vi "纳清蓝绿藻电极校准.vi"() -> ()   [LabVIEW 2016, in "斯坦道多参数.lvlib"]
uses:
  <vilib>/Utility/miscctls.llb/LVPointTypeDef.ctl
  <vilib>/Utility/miscctls.llb/LVPositionTypeDef.ctl
  <vilib>/Analysis/NI_AALBase.lvlib
panel:
  out "滤波设定":sgl
  in  "量程":u16(ring) items=["0-2000000", "0-200000"]
  out "第三点信号值":dbl
  out "第二点信号值":dbl
  out "第一点信号值":dbl
  out "报警信息":string
  out "通讯状态":string
  out "第三点校准值":dbl
  out "标液3":sgl
  out "第二点校准值":dbl
  out "第一点校准值":dbl
  in  "校准停止":bool
  in  "校准启动":bool
  in  "校准模式":u16(ring)=1 items=["两点校准", "单点校准", "三点校准"]
  out "最小值":sgl format="%#.2f"
  out "最大值":sgl format="%#.2f"
  out "波形图表":dbl(graph) caption="历史曲线"
  out "mean":dbl caption="均值" format="%#.2f"
  out "standard deviation":dbl caption="标准差" format="%#.2f"
  out "变异系数":dbl format="%#.6f"
  out "测量值":sgl format="%#.2f"
  out "提示":string
  out "标液2":sgl
  out "标液1":sgl
  out "原始光强数值":u16 caption="信号值"
  out "温度":dbl format="%#.2f"
  # "藻密度电极设定"
  # "℃"
  # "cells/mL"
  # "cells/mL"
  # "请选择校准模式:"
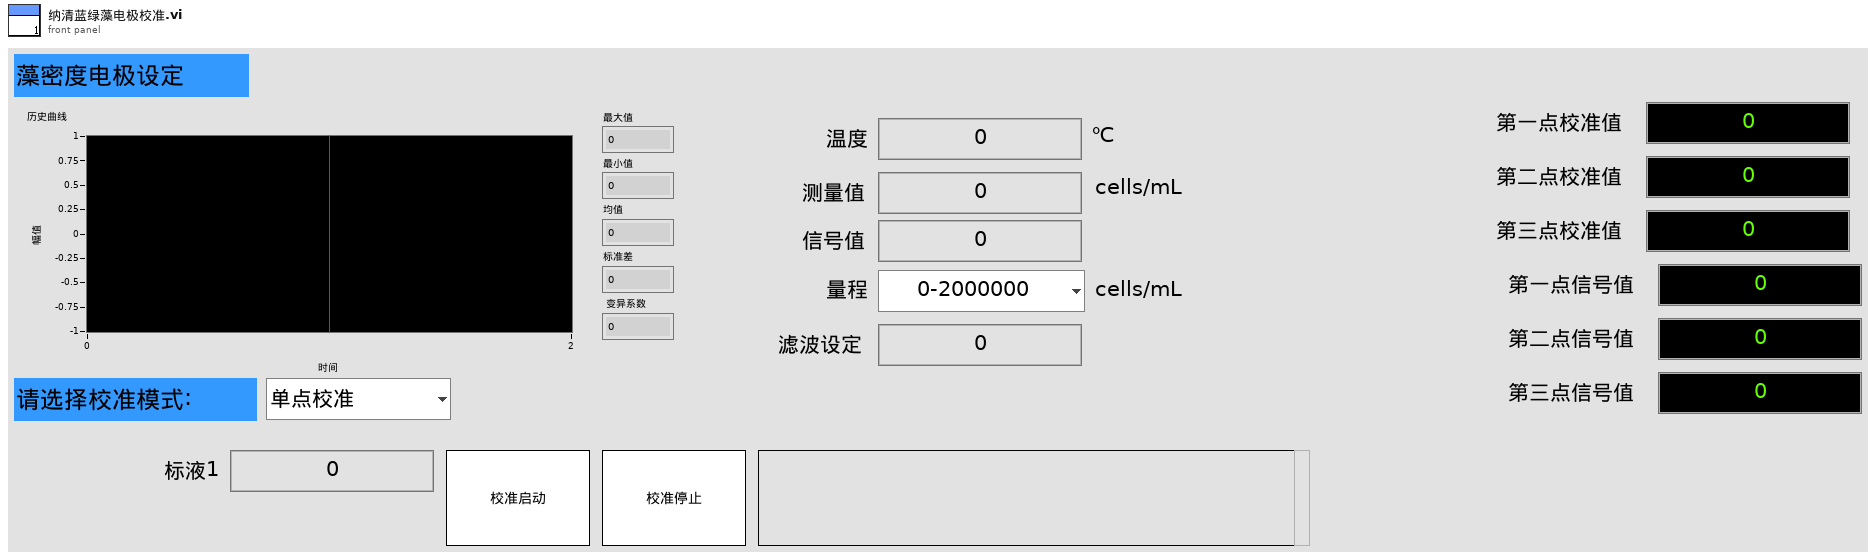
[diagram p1: front panel]
types:
  T1 = typedef "LVPointTypeDef.ctl" = cluster{"Horizontal":i16, "Vertical":i16}
  T2 = cluster{"报警码":u16, "蓝绿藻":sgl, "温度数据":sgl, "原始光强数值":u16, "量程":u16, "平均次数":u16, "清扫模式":u16, "清扫次数":u16, "清扫间隔分钟":u16, "0X000B_NC":string, "产品名称":string, "序列号":string, "硬件版本":string, "软件版本":string, "通讯地址":u16, "波特率":u16, "设备类型":u16, "0X0026_NC":string, "校准量程":u16, "第一点原始光强":u16, "第一点校准数据":sgl, "第二点原始光强":u16, "第二点校准数据":sgl, "第三点原始光强":u16, "第三点校准数据":sgl, "探头校准命令":u16, "温度校准参数":sgl, "温度校准命令":u16}
  T3 = cluster{"pH":u32, "DO":u32, "Cond":u32, "Turb":u32, "叶绿素a":u32, "藻密度":u32, "ORP":u32}
  T4 = typedef "LVPositionTypeDef.ctl" = cluster{"Left":i32, "Top":i32}
  T5 = enum8{"Enabled", "Disabled", "Disabled and Grayed Out"}
  T6 = cluster{"报警码":u16, "蓝绿藻":sgl, "温度数据":sgl, "原始光强数值":u16, "0X0006_NC":u16, "平均次数":u16, "清扫模式":u16, "清扫次数":u16, "清扫间隔分钟":u16, "0X000B_NC":string, "产品名称":string, "序列号":string, "硬件版本":string, "软件版本":string, "通讯地址":u16, "波特率":u16, "设备类型":u16, "0X0026_NC":string, "0X0030_NC":u16, "第一点原始光强":u16, "第一点校准数据":sgl, "第二点原始光强":u16, "第二点校准数据":sgl, "第三点原始光强":u16, "第三点校准数据":sgl, "探头校准命令":u16, "温度校准参数":sgl, "温度校准命令":u16}
  T7 = cluster{"ph":bool, "DO":bool, "Cond":bool, "Turb":bool, "叶绿素a":bool, "藻密度":bool, "ORP":bool}
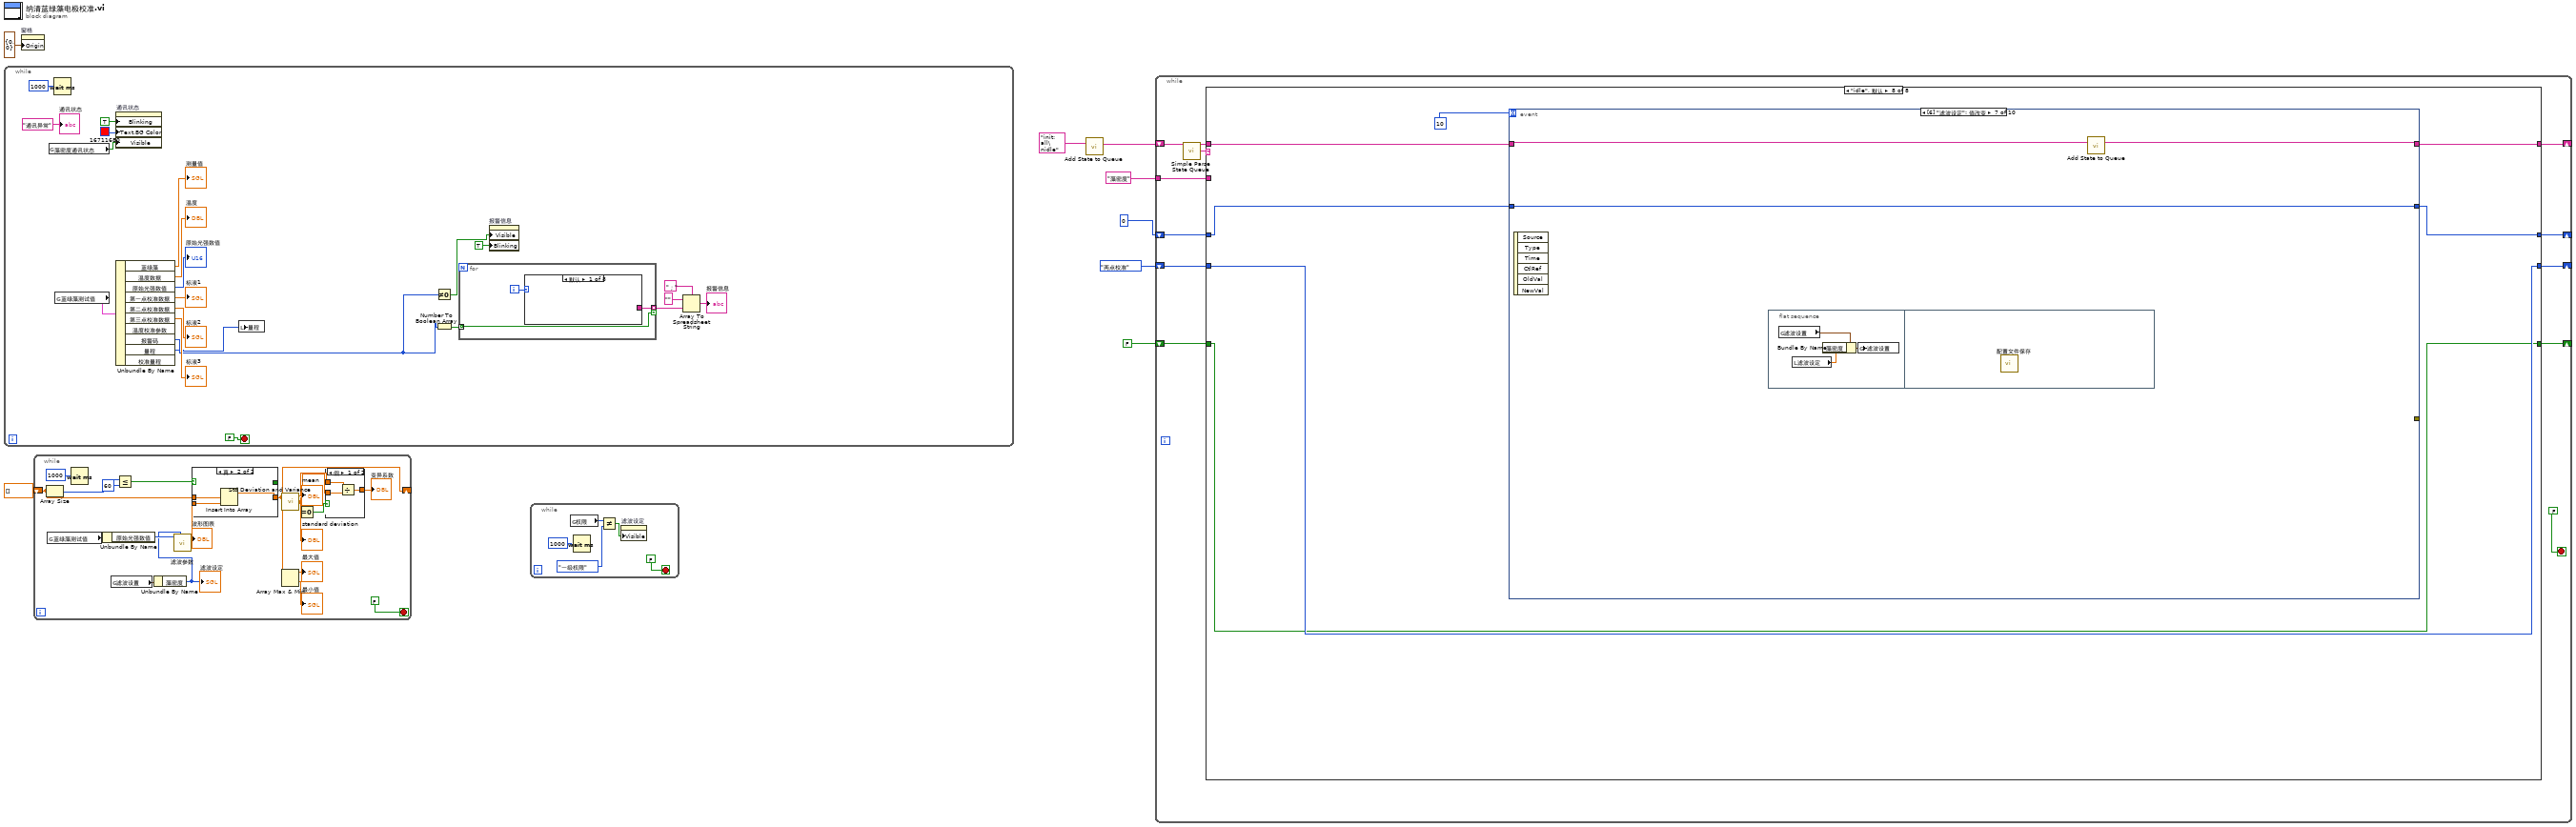
[diagram p0: block diagram]
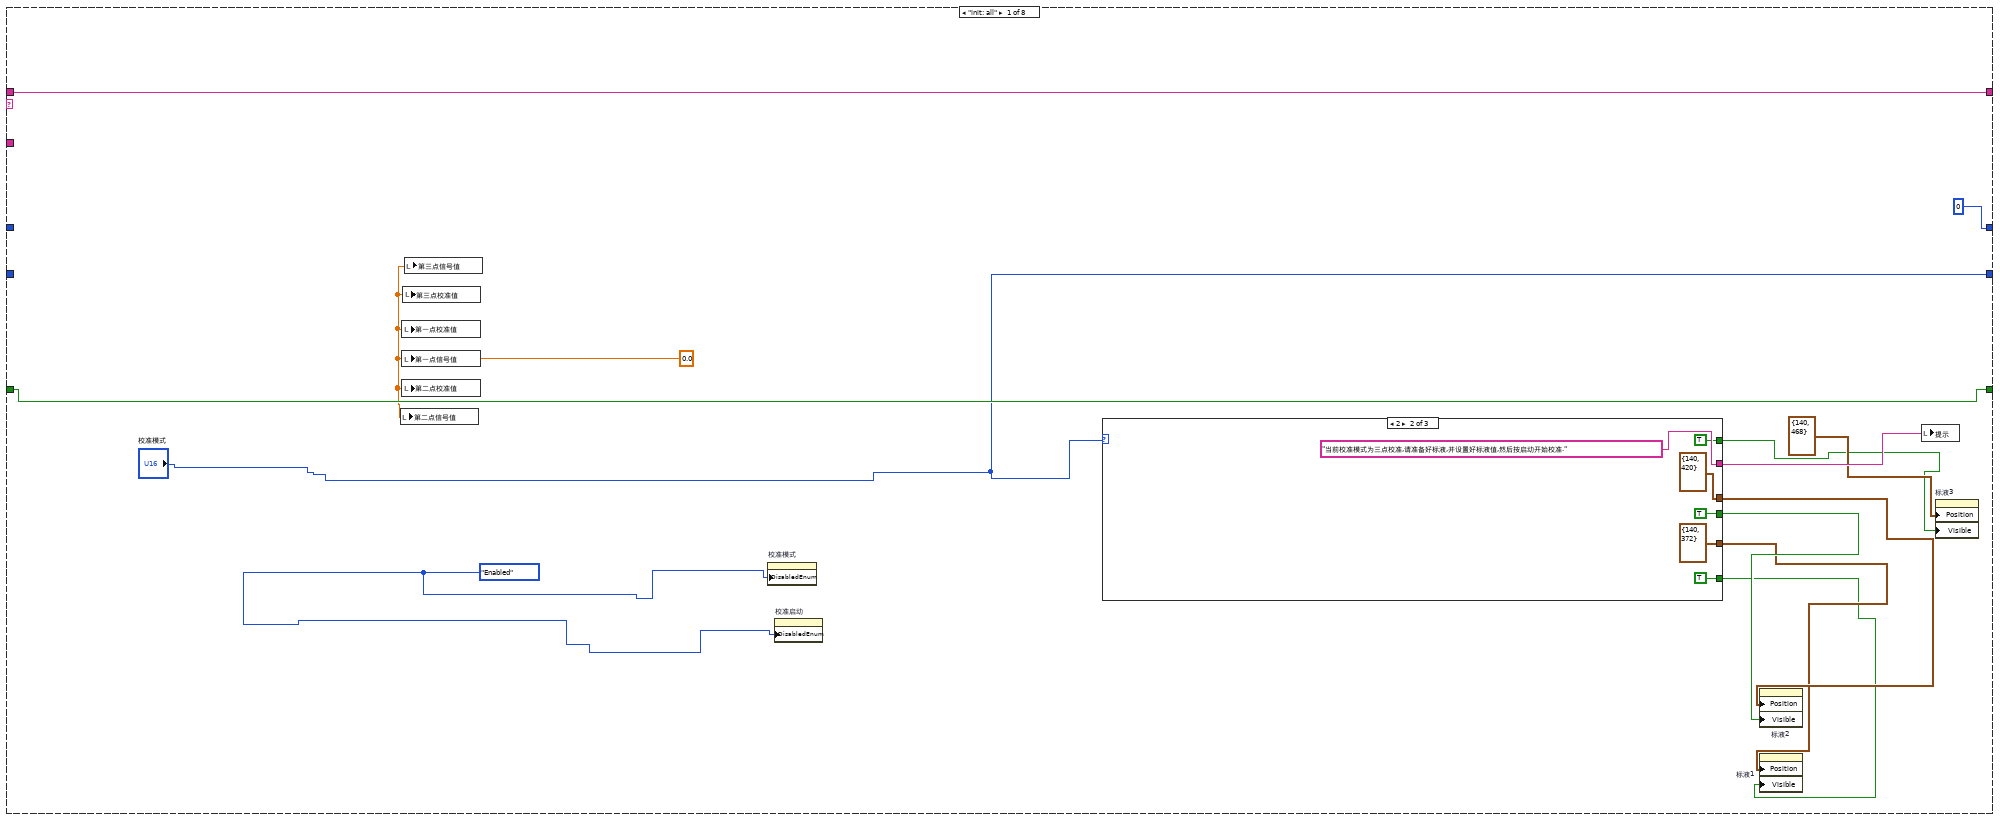
[diagram p2: hidden frame]
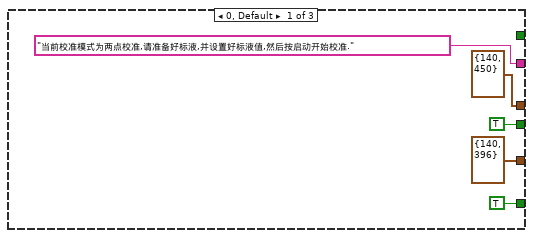
[diagram p3: hidden frame]
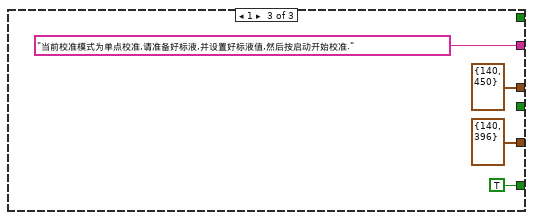
[diagram p4: hidden frame]
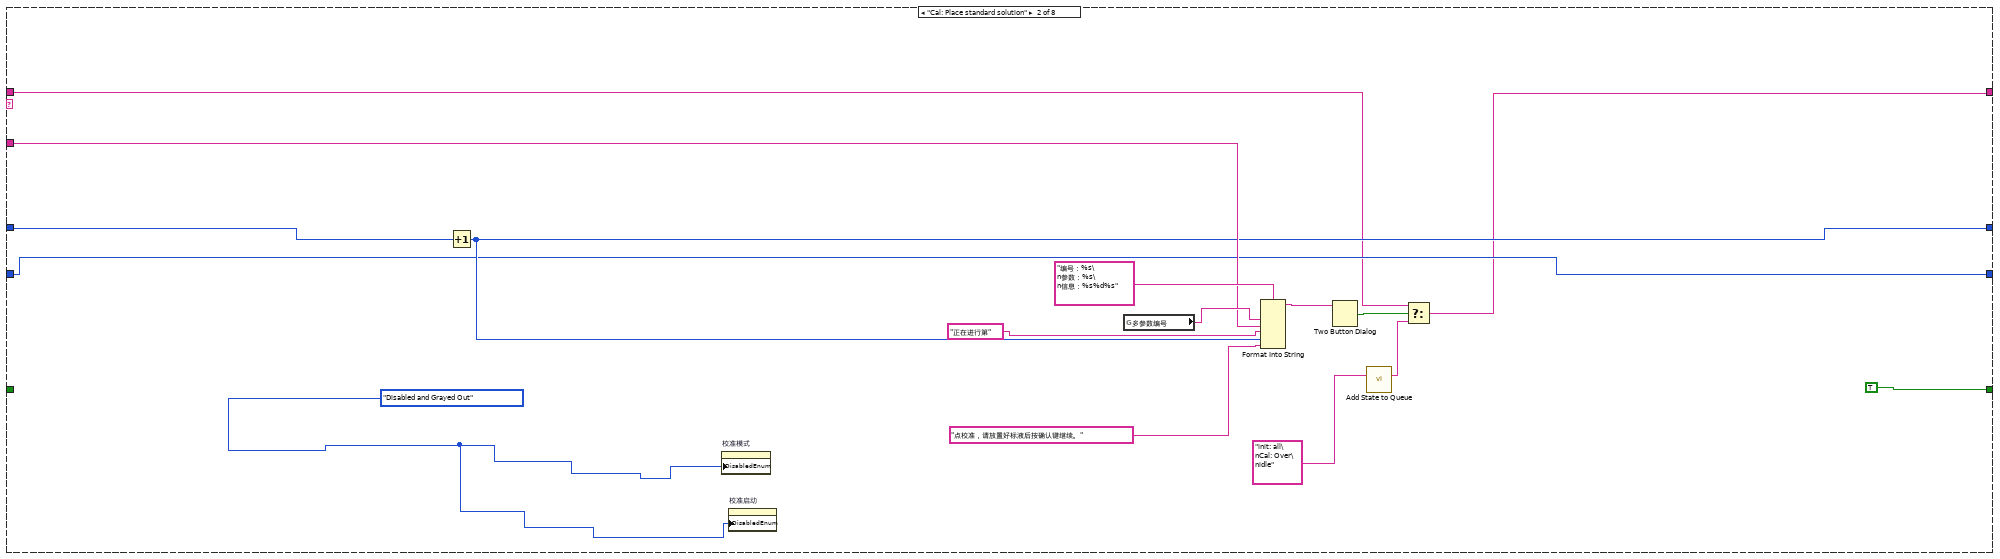
[diagram p5: hidden frame]
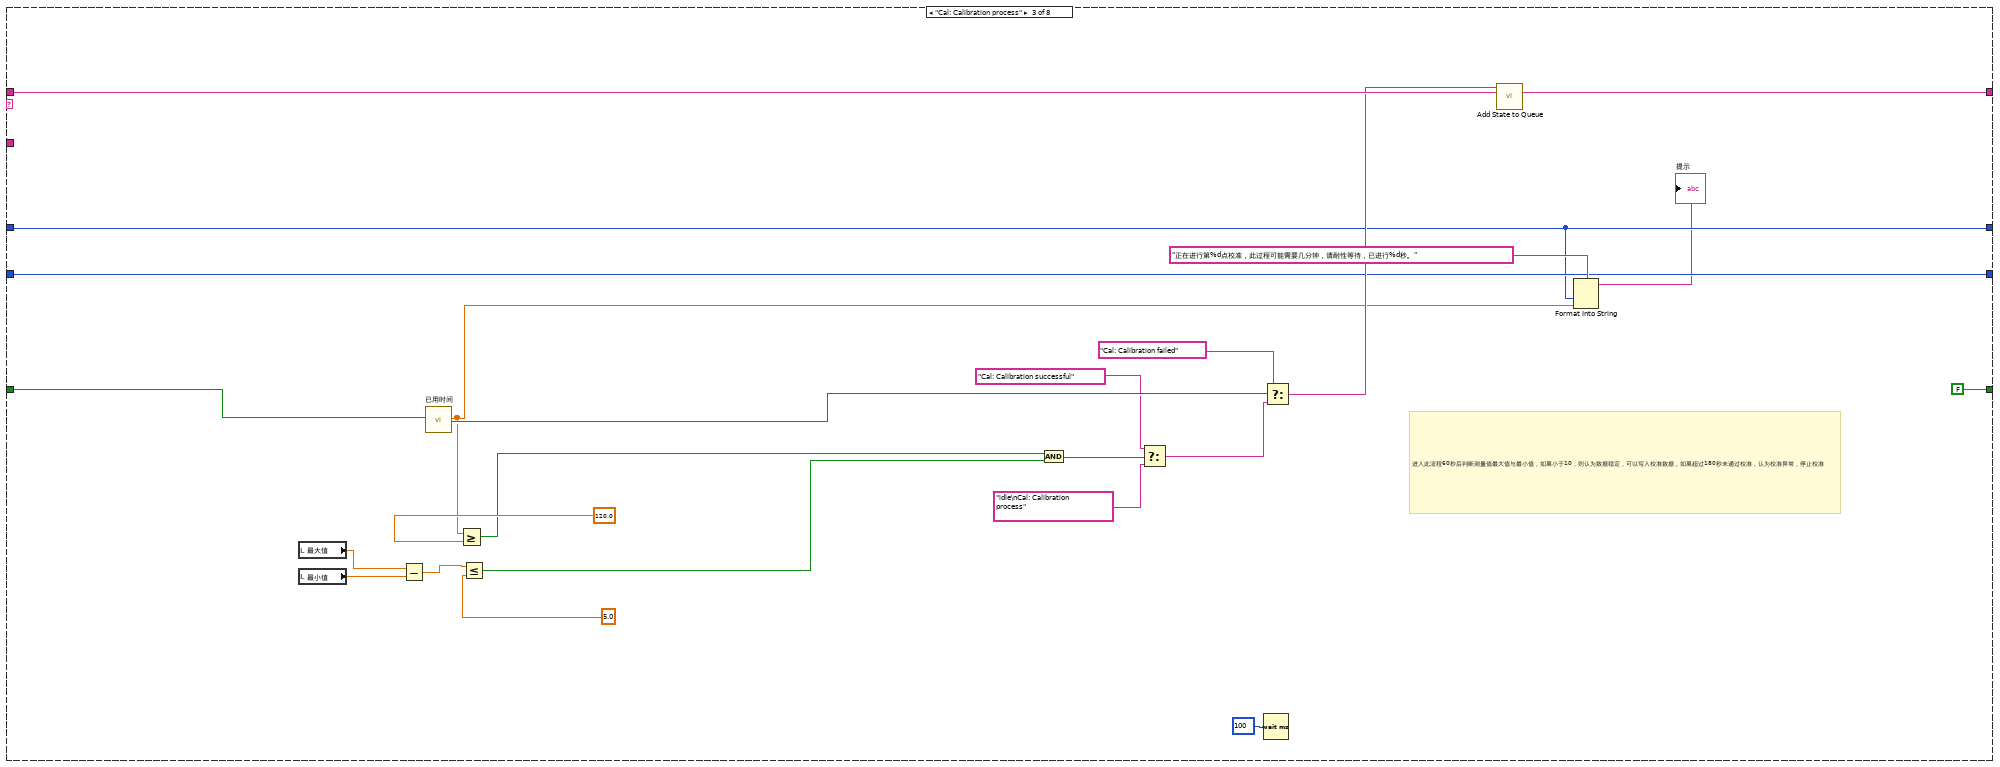
[diagram p6: hidden frame]
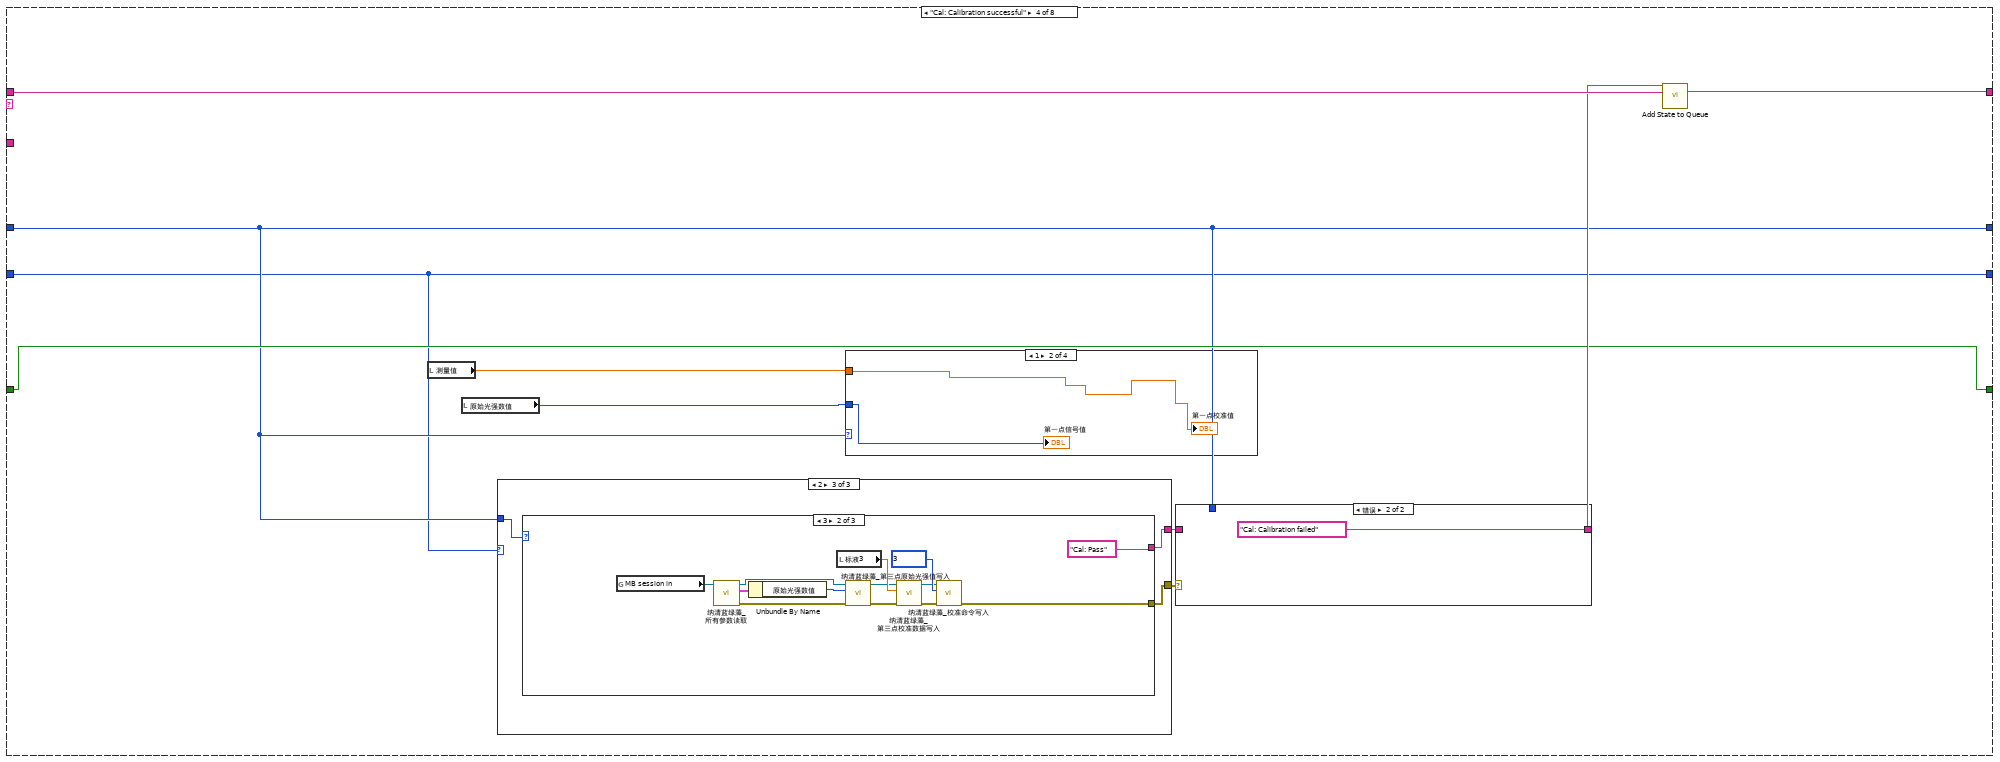
[diagram p7: hidden frame]
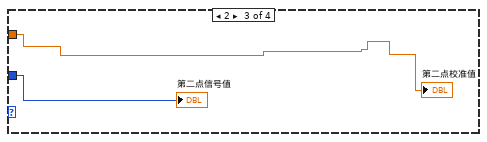
[diagram p9: hidden frame]
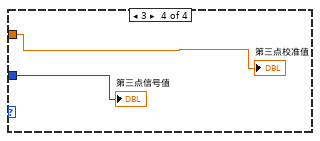
[diagram p10: hidden frame]
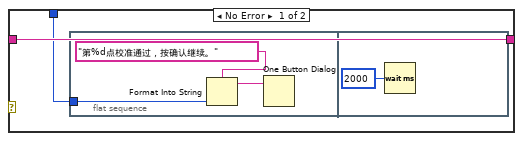
[diagram p11: hidden frame]
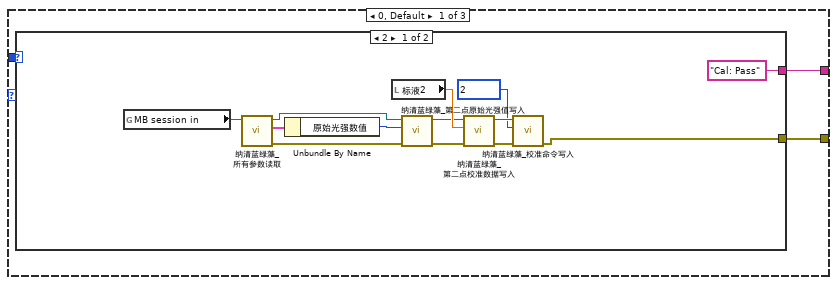
[diagram p12: hidden frame]
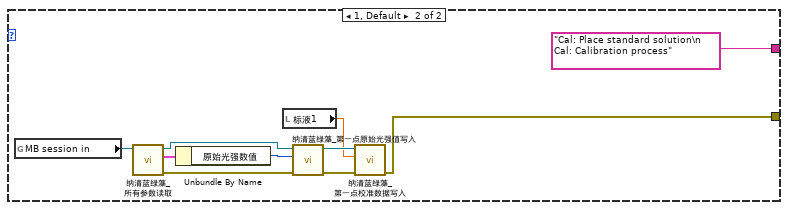
[diagram p13: hidden frame]
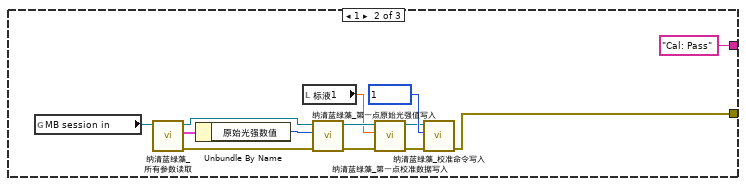
[diagram p14: hidden frame]
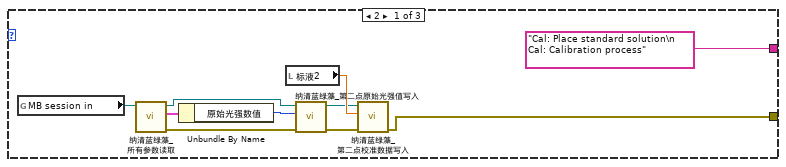
[diagram p15: hidden frame]
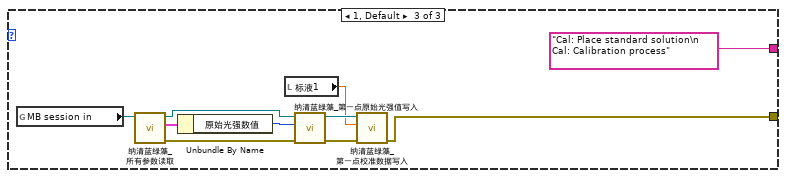
[diagram p16: hidden frame]
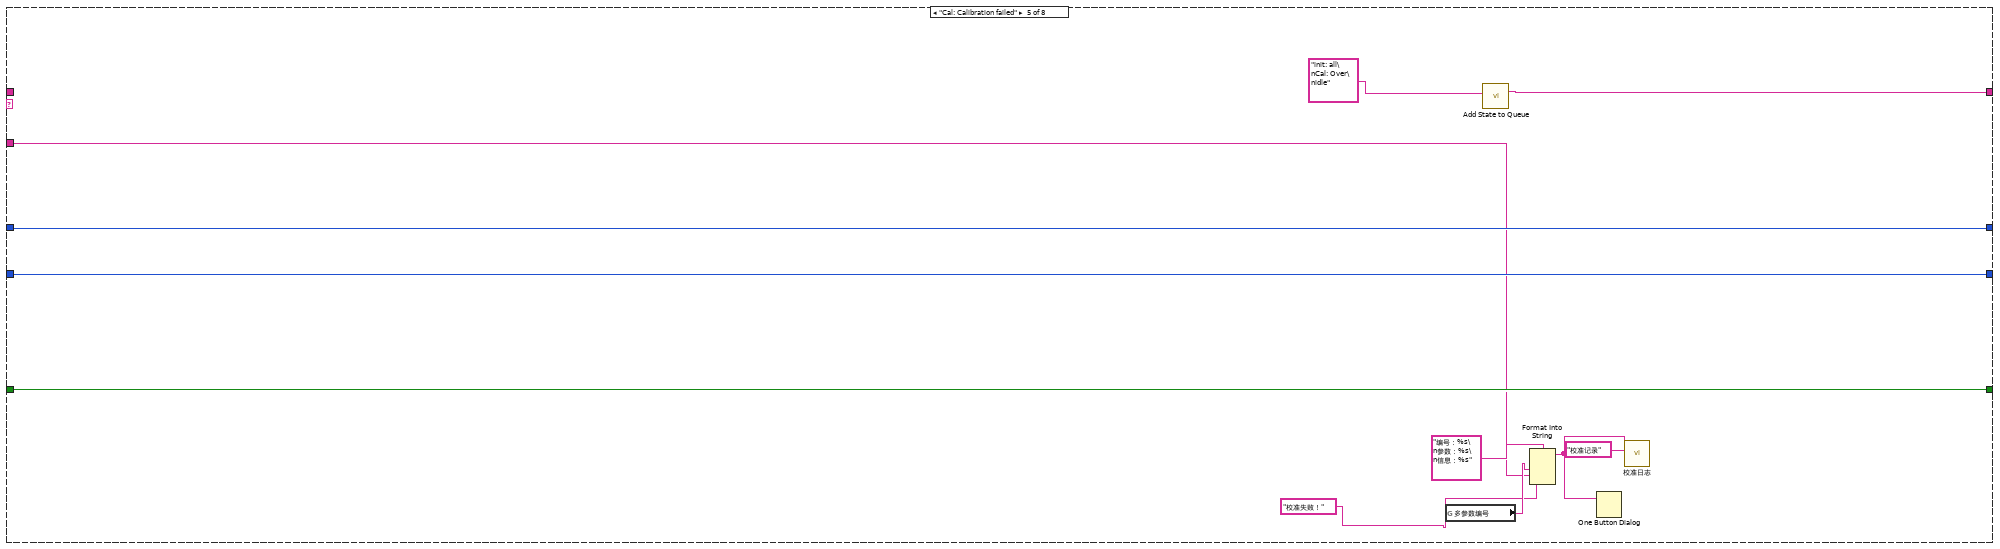
[diagram p17: hidden frame]
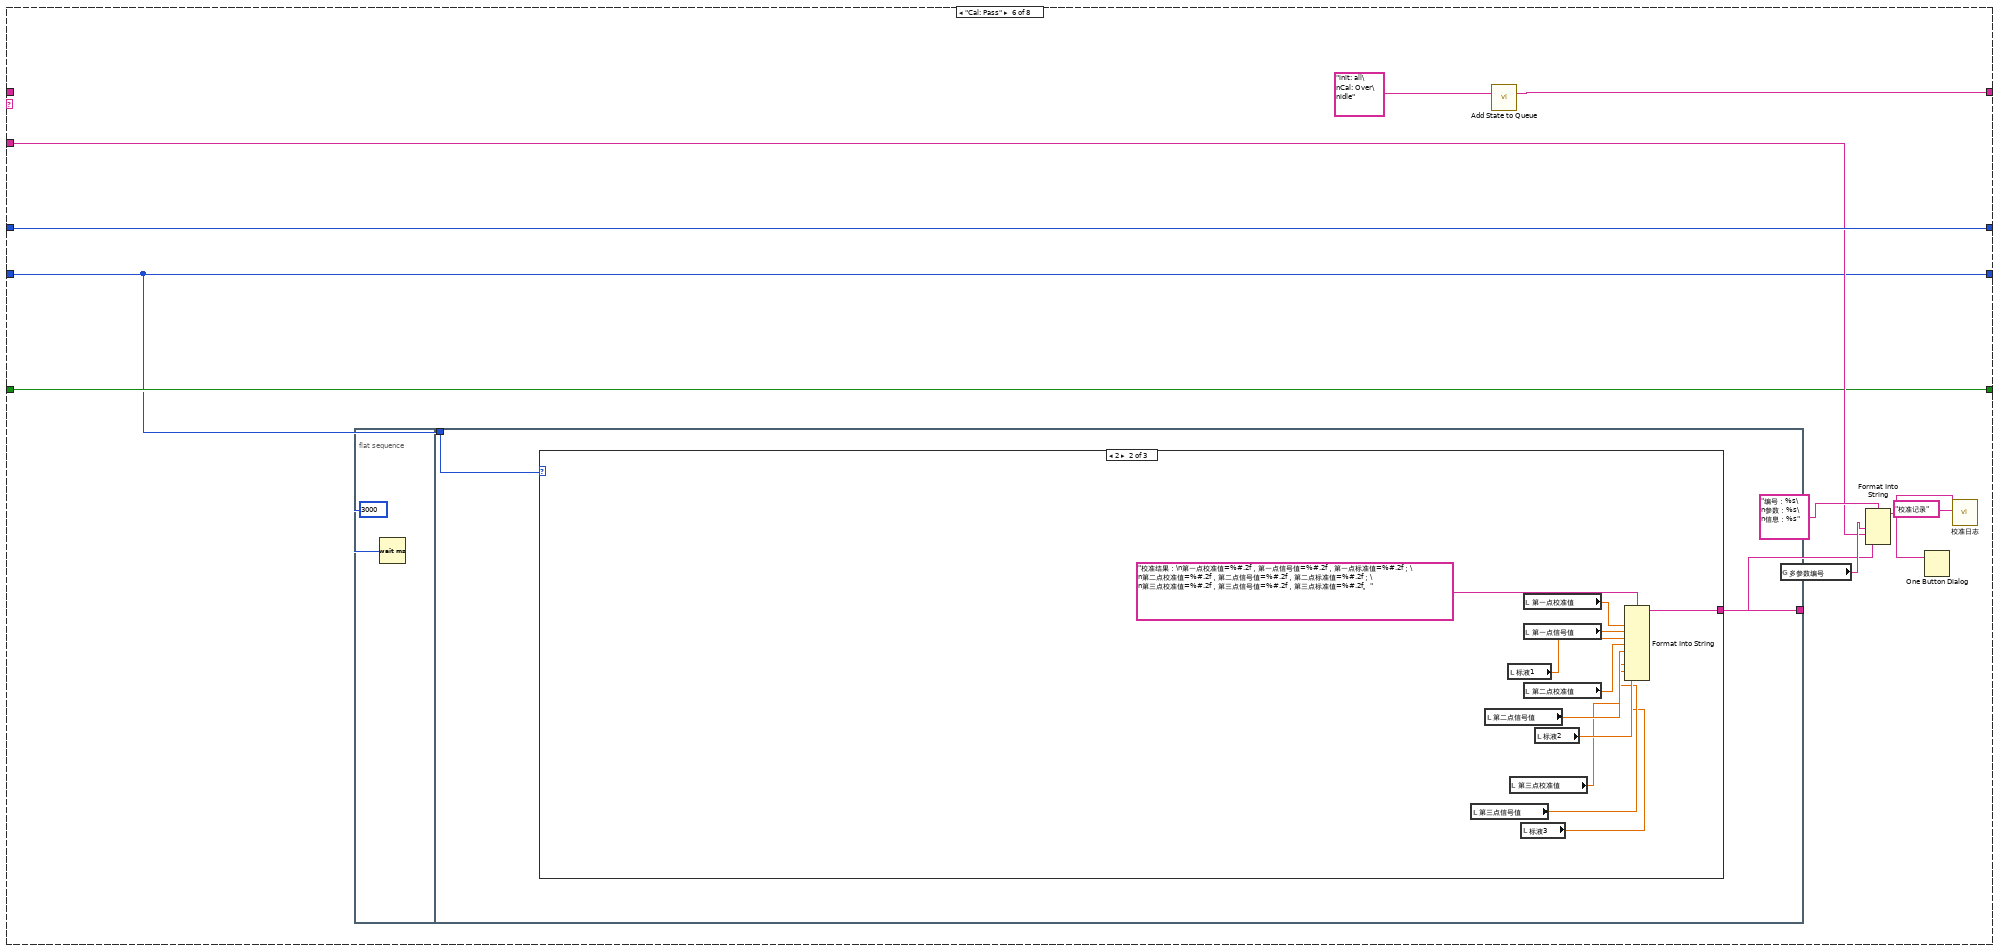
[diagram p18: hidden frame]
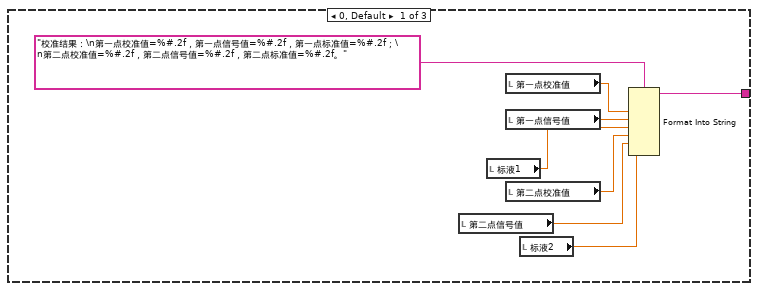
[diagram p19: hidden frame]
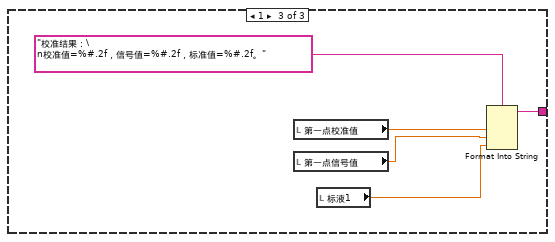
[diagram p20: hidden frame]
diagram:
  n1 = while {
    stop <- FALSE stop-if-true
    n2 = global read "多参数全局变量.vi" "藻密度通讯状态"() -> (w18:bool)
    n3 = Wait (ms)(milliseconds to wait=u32 1000 ("等待时间（毫秒）")) -> ()  [unwired: 1 out]
    n4 = global read "纳清过程全局变量.vi" "蓝绿藻测试值"() -> (w28:T2)
    n5 = property on="通讯状态" class="Str"("Blinking"=TRUE ("闪烁"), "Text.BG Color"=u32 16711680, "Visible"=w18) -> ()  [unwired: 2 in, 2 out]
    n6 = Unbundle By Name(w28) -> ("蓝绿藻"=→"测量值":sgl, "温度数据"=→"温度":sgl, "原始光强数值"=→"原始光强数值":u16, "第一点校准数据"=→"标液1":sgl, "第二点校准数据"=→"标液2":sgl, "第三点校准数据"=→"标液3":sgl, "报警码"=w10:u16, "量程"=w9:u16)  [unwired: 2 out]
    n7 = local write "量程"(w9) -> ()
    n8 = Not Equal To 0?(x=w10) -> (x != 0?=w12:bool)
    n9 = Number To Boolean Array(number=w10) -> (Boolean array=w17:bool[])
    n10 = for {
      tunnel: w17 -> [w31] mode=indexing
      tunnel: [w32] -> w16 mode=indexing if=w31
      i -> [w33]
      n11 = case shown="默认" w33 {
        tunnel: [_ "测量值超量程" "温度超量程" "光强信号超范围" "清扫中" "温度传感器故障" "电极故障" "内部电压基准故障"] -> w32
        frame Default {
        }
        frame 0 {
        }
        frame 2 {
        }
        frame 3 {
        }
        frame 4 {
        }
        frame 8 {
        }
        frame 9 {
        }
        frame 10 {
        }
      }
    }
    n12 = property on="报警信息" class="Str"("Visible"=w12, "Blinking"=TRUE ("闪烁")) -> ()  [unwired: 2 in, 2 out]
    n13 = Array To Spreadsheet String(delimiter (Tab)="；" ("分隔符(Tab)"), array=w16, 3:"" ("格式字符串")) -> (spreadsheet string=→"报警信息":string)
    "通讯状态" <- "通讯异常" ("当前串口")
  }
  n14 = property on="窗格" class="Pane"("Origin"=T1 {"Horizontal"=0, "Vertical"=0} ("原点")) -> ()  [unwired: 2 in, 2 out]
  n15 = while {
    shift-right: [w48] -> _
    shift-left: sgl[] [] -> [w54]
    stop <- FALSE stop-if-true
    n16 = Array Size(array=w54) -> (size(s)=w56:i32)
    n17 = global read "纳清过程全局变量.vi" "蓝绿藻测试值"() -> (w45:T2)
    n18 = Wait (ms)(milliseconds to wait=u32 1000 ("等待时间（毫秒）")) -> ()  [unwired: 1 out]
    n19 = Unbundle By Name(w45) -> ("原始光强数值"=w44:u16)
    n20 = global read "断电保存变量.vi" "滤波设置"() -> (w42:T3)
    n21 = Less Or Equal?(x=w56, y=60) -> (x <= y?=w55:bool)
    n22 = Unbundle By Name(w42) -> ("藻密度"=w41:u32)
    "滤波设定" <- w41
    n23 = call "滤波参数.vi"("滤波次数"=w41, "x"=w44) -> ("mode"=w43:dbl)  [unwired: 9 in]
    "波形图表" <- w43
    n24 = case shown="真" w55 {
      tunnel: w54 -> [w67 w70]
      tunnel: w43 -> [w65 w69]
      tunnel: [w63 w68] -> w48
      tunnel: [TRUE _] -> _
      frame False {
        n25 = Replace Array Subset(array=w67, new element=w65) -> (w66:sgl[])  [unwired: 1 in]
        n26 = Rotate 1D Array(1:w66, 2:-1 ("n")) -> (0:w63:sgl[])
      }
      frame True {
        n27 = Insert Into Array(array=w70, new element=w69) -> (w68:sgl[])  [unwired: 1 in]
      }
    }
    n28 = call <vilib>:"Std Deviation and Variance.vi"("X"=w48) -> ("mean"=w52:dbl, "standard deviation"=w51:dbl)  [unwired: 1 in, 1 out]
    "mean" <- w52
    "standard deviation" <- w51
    n29 = Array Max & Min(array=w48) -> (max value=→"最大值":sgl, min value=→"最小值":sgl)  [unwired: 2 out]
    n30 = Equal To 0?(x=w52) -> (x = 0?=w53:bool)
    n31 = case shown="假" w53 {
      tunnel: w51 -> [w61 _]
      tunnel: [w60 _] -> w50
      tunnel: w52 -> [w59 _]
      frame False {
        n32 = Divide(x=w61, y=w59) -> (x/y=w60:dbl)
      }
      frame True {
      }
    }
    "变异系数" <- w50
  }
  n33 = while {
    stop <- FALSE stop-if-true
    n34 = global read "多参数全局变量.vi" "权限"() -> (w74:enum16{"一级权限", "二级权限", "三级权限"})
    n35 = Wait (ms)(milliseconds to wait=u32 1000 ("等待时间（毫秒）")) -> ()  [unwired: 1 out]
    n36 = Not Equal?(x=w74, y=enum16{"一级权限", "二级权限", "三级权限"}."一级权限") -> (x != y?=w71:bool)
    n37 = property on="滤波设定" class="DigNum (严格)"("Visible"=w71) -> ()  [unwired: 2 in, 2 out]
  }
  n38 = call "Add State to Queue.vi"("State(s) In (\"\")"="init: all\nidle" ("State(s) In (\"\")")) -> ("States Out"=w5:string)  [unwired: 14 in]
  n39 = while {
    shift-right: [w83] -> _
    shift-left: w5 -> [w87]
    shift-right: [w80] -> _
    shift-left: 0 -> [w82]
    tunnel: "藻密度" ("State(s) In (\"\")") -> [w81]
    shift-right: [w78] -> _
    shift-left: enum16{"两点校准", "单点校准", "三点校准"}."两点校准" ("校准模式") -> [w79]
    shift-right: [w76] -> _
    shift-left: FALSE -> [w77]
    stop <- FALSE stop-if-true
    n40 = call "Simple Parse State Queue.vi"("State Queue"=w87) -> ("Remain States"=w84:string, "Next State"=w85:string)  [unwired: 13 in]
    n41 = case shown="\"idle\", 默认" w85 {
      tunnel: w84 -> [w100 w119 w150 w163 _ _ w306 w316]
      tunnel: [w100 w118 w149 w162 w261 w266 w306 w315] -> w83
      tunnel: w82 -> [_ w127 w134 w157 w264 w275 w305 w313]
      tunnel: w81 -> [_ w128 _ _ w255 w271 _ _]
      tunnel: [0 w125 w134 w157 w264 w275 w305 w314] -> w80
      tunnel: w79 -> [_ w124 w135 w156 w263 w267 w304 w312]
      tunnel: ["校准模式" w124 w135 w156 w263 w267 w304 w312] -> w78
      tunnel: w77 -> [w98 _ w137 w158 w262 w270 w303 w310]
      tunnel: [w98 TRUE FALSE w158 w262 w270 w303 w310] -> w76
      frame "init: all" {
        w94 = T5."Enabled" ("禁用")
        w97 = 0.0 ("第一点校准值")
        n42 = local write "第二点信号值"(w97) -> ()
        n43 = local write "第一点校准值"(w97) -> ()
        n44 = local write "第一点信号值"(w97) -> ()
        n45 = local write "第二点校准值"(w97) -> ()
        n46 = local write "第三点校准值"(w97) -> ()
        n47 = local write "第三点信号值"(w97) -> ()
        n48 = property on="校准模式" class="Ring (严格)"("DisabledEnum"=w94) -> ()  [unwired: 2 in, 2 out]
        n49 = property on="校准启动" class="Bool"("DisabledEnum"=w94) -> ()  [unwired: 2 in, 2 out]
        n50 = case shown="2" "校准模式" {
          tunnel: ["当前校准模式为两点校准,请准备好标液,并设置好标液值,然后按启动开始校准." ("提示") "当前校准模式为三点校准,请准备好标液,并设置好标液值,然后按启动开始校准." ("提示") "当前校准模式为单点校准,请准备好标液,并设置好标液值,然后按启动开始校准." ("提示")] -> w96
          tunnel: [TRUE ("可见") TRUE ("可见") _] -> w90
          tunnel: [T4 {"Left"=140, "Top"=396} ("位置") T4 {"Left"=140, "Top"=372} ("位置") T4 {"Left"=140, "Top"=396} ("位置")] -> w89
          tunnel: [T4 {"Left"=140, "Top"=450} ("位置 2") T4 {"Left"=140, "Top"=420} ("位置 2") T4 {"Left"=140, "Top"=450} ("位置 2")] -> w91
          tunnel: [_ TRUE ("可见") _] -> w92
          tunnel: [TRUE ("可见") TRUE ("可见") TRUE ("可见")] -> w88
          frame 0, Default {
          }
          frame 2 {
          }
          frame 1 {
          }
        }
        n51 = property on="标液2" class="DigNum (严格)"("Position"=w91, "Visible"=w90) -> ()  [unwired: 2 in, 2 out]
        n52 = property on="标液1" class="DigNum (严格)"("Position"=w89, "Visible"=w88) -> ()  [unwired: 2 in, 2 out]
        n53 = local write "提示"(w96) -> ()
        n54 = property on="标液3" class="DigNum (严格)"("Position"=T4 {"Left"=140, "Top"=468} ("位置 3"), "Visible"=w92) -> ()  [unwired: 2 in, 2 out]
      }
      frame "Cal: Place standard solution" {
        w117 = T5."Disabled and Grayed Out" ("禁用")
        n55 = Increment(x=w127) -> (x+1=w125:i32)
        n56 = property on="校准模式" class="Ring (严格)"("DisabledEnum"=w117) -> ()  [unwired: 2 in, 2 out]
        n57 = property on="校准启动" class="Bool"("DisabledEnum"=w117) -> ()  [unwired: 2 in, 2 out]
        n58 = global read "多参数全局变量.vi" "多参数编号"() -> (w130:string)
        n59 = Format Into String(format string="编号：%s\n参数：%s\n信息：%s%d%s" ("格式字符串"), w130, w128, "正在进行第" ("消息"), w125, "点校准，请放置好标液后按确认键继续。" ("消息")) -> (resulting string=w122:string)  [unwired: 2 in, 1 out]
        n60 = Two Button Dialog(message=w122) -> (T button?=w121:bool)  [unwired: 2 in]
        n61 = call "Add State to Queue.vi"("State(s) In (\"\")"="init: all\nCal: Over\nidle" ("State(s) In (\"\")")) -> ("States Out"=w120:string)  [unwired: 14 in]
        n62 = Select(t=w119, s=w121, f=w120) -> (s? t:f=w118:string)
      }
      frame "Cal: Calibration process" {
        # "进入此流程60秒后判断测量值最大值与最小值，如果小于10，则认为数据稳定，可以写入校准数据，如果超过180秒未通过校准，认为校准异常，停止校准"
        n63 = local read "最大值"() -> (w154:sgl)
        n64 = local read "最小值"() -> (w153:sgl)
        n65 = Subtract(x=w154, y=w153) -> (x-y=w155:sgl)
        n66 = call "已用时间"("Reset"=w137) -> ("Elapsed Time (s)"=w133:dbl, "Time has Elapsed"=w151:bool)  [unwired: 11 in, 6 out]
        n67 = Greater Or Equal?(x=w133, y=120.0) -> (x >= y?=w146:bool)
        n68 = Less Or Equal?(x=w155, y=5.0) -> (x <= y?=w142:bool)
        n69 = And(x=w146, y=w142) -> (x .and. y?=w143:bool)
        n70 = Select(t="Cal: Calibration successful" ("State(s) In (\"\")"), s=w143, f="idle\nCal: Calibration process" ("State(s) In (\"\")")) -> (s? t:f=w141:string)
        n71 = Wait (ms)(milliseconds to wait=u32 100 ("等待时间（毫秒）")) -> ()  [unwired: 1 out]
        n72 = Select(t="Cal: Calibration failed" ("State(s) In (\"\")"), s=w151, f=w141) -> (s? t:f=w140:string)
        n73 = call "Add State to Queue.vi"("State(s) In Front (\"\")"=w140, "State(s) In (\"\")"=w150) -> ("States Out"=w149:string)  [unwired: 13 in]
        n74 = Format Into String(format string="正在进行第%d点校准，此过程可能需要几分钟，请耐性等待，已进行%d秒。" ("格式字符串"), w134, w133) -> (resulting string=→"提示":string)  [unwired: 2 in, 1 out]
      }
      frame "Cal: Calibration successful" {
        n75 = local read "测量值"() -> (w159:sgl)
        n76 = local read "原始光强数值"() -> (w160:u16)
        n77 = case shown="2" w156 {
          tunnel: [w181 w205 w218] -> w165
          tunnel: [w180 "Cal: Pass" ("State(s) In (\"\")") w219] -> w164
          tunnel: w157 -> [w179 _ w220]
          frame 0, Default {
            n78 = case shown="2" w179 {
              tunnel: [w182 w195] -> w181
              tunnel: ["Cal: Pass" ("State(s) In (\"\")") "Cal: Place standard solution\n Cal: Calibration process" ("State(s) In (\"\")")] -> w180
              frame 2 {
                n79 = global read "多参数全局变量.vi" "MB session in"() -> (w186:refnum<class "MB_Master.lvclass">)
                n80 = call "纳清蓝绿藻_所有参数读取.vi"("MB session in"=w186) -> ("error out"=w184:errorcluster, "输出值"=w187:T6, "MB session out"=w185:refnum<class "MB_Master.lvclass">)  [unwired: 8 in]
                n81 = Unbundle By Name(w187) -> ("原始光强数值"=w188:u16)
                n82 = local read "标液2"() -> (w193:sgl)
                n83 = call "纳清蓝绿藻_第二点原始光强值写入.vi"("error in (no error)"=w184, "数值"=w188, "MB session in"=w185) -> ("error out"=w189:errorcluster, "MB session out"=w190:refnum<class "MB_Master.lvclass">)  [unwired: 7 in]
                n84 = call "纳清蓝绿藻_第二点校准数据写入.vi"("error in (no error)"=w189, "数值"=w193, "MB session in"=w190) -> ("error out"=w191:errorcluster, "MB session out"=w192:refnum<class "MB_Master.lvclass">)  [unwired: 7 in]
                n85 = call "纳清蓝绿藻_校准命令写入.vi"("error in (no error)"=w191, "数值"=u16 2 ("starting address"), "MB session in"=w192) -> ("error out"=w182:errorcluster)  [unwired: 7 in, 1 out]
              }
              frame 1, Default {
                n86 = global read "多参数全局变量.vi" "MB session in"() -> (w201:refnum<class "MB_Master.lvclass">)
                n87 = call "纳清蓝绿藻_所有参数读取.vi"("MB session in"=w201) -> ("error out"=w203:errorcluster, "输出值"=w200:T6, "MB session out"=w202:refnum<class "MB_Master.lvclass">)  [unwired: 8 in]
                n88 = Unbundle By Name(w200) -> ("原始光强数值"=w199:u16)
                n89 = local read "标液1"() -> (w196:sgl)
                n90 = call "纳清蓝绿藻_第一点原始光强值写入.vi"("error in (no error)"=w203, "数值"=w199, "MB session in"=w202) -> ("error out"=w198:errorcluster, "MB session out"=w197:refnum<class "MB_Master.lvclass">)  [unwired: 7 in]
                n91 = call "纳清蓝绿藻_第一点校准数据写入.vi"("error in (no error)"=w198, "数值"=w196, "MB session in"=w197) -> ("error out"=w195:errorcluster)  [unwired: 7 in, 1 out]
              }
            }
          }
          frame 1 {
            n92 = global read "多参数全局变量.vi" "MB session in"() -> (w213:refnum<class "MB_Master.lvclass">)
            n93 = call "纳清蓝绿藻_所有参数读取.vi"("MB session in"=w213) -> ("error out"=w215:errorcluster, "输出值"=w212:T6, "MB session out"=w214:refnum<class "MB_Master.lvclass">)  [unwired: 8 in]
            n94 = Unbundle By Name(w212) -> ("原始光强数值"=w211:u16)
            n95 = local read "标液1"() -> (w206:sgl)
            n96 = call "纳清蓝绿藻_第一点原始光强值写入.vi"("error in (no error)"=w215, "数值"=w211, "MB session in"=w214) -> ("error out"=w210:errorcluster, "MB session out"=w209:refnum<class "MB_Master.lvclass">)  [unwired: 7 in]
            n97 = call "纳清蓝绿藻_第一点校准数据写入.vi"("error in (no error)"=w210, "数值"=w206, "MB session in"=w209) -> ("error out"=w208:errorcluster, "MB session out"=w207:refnum<class "MB_Master.lvclass">)  [unwired: 7 in]
            n98 = call "纳清蓝绿藻_校准命令写入.vi"("error in (no error)"=w208, "数值"=u16 1 ("starting address"), "MB session in"=w207) -> ("error out"=w205:errorcluster)  [unwired: 7 in, 1 out]
          }
          frame 2 {
            n99 = case shown="3" w220 {
              tunnel: [w221 w231 w244] -> w218
              tunnel: ["Cal: Place standard solution\n Cal: Calibration process" ("State(s) In (\"\")") "Cal: Pass" ("State(s) In (\"\")") "Cal: Place standard solution\n Cal: Calibration process" ("State(s) In (\"\")")] -> w219
              frame 2 {
                n100 = global read "多参数全局变量.vi" "MB session in"() -> (w224:refnum<class "MB_Master.lvclass">)
                n101 = call "纳清蓝绿藻_所有参数读取.vi"("MB session in"=w224) -> ("error out"=w222:errorcluster, "输出值"=w225:T6, "MB session out"=w223:refnum<class "MB_Master.lvclass">)  [unwired: 8 in]
                n102 = Unbundle By Name(w225) -> ("原始光强数值"=w226:u16)
                n103 = local read "标液2"() -> (w229:sgl)
                n104 = call "纳清蓝绿藻_第二点原始光强值写入.vi"("error in (no error)"=w222, "数值"=w226, "MB session in"=w223) -> ("error out"=w227:errorcluster, "MB session out"=w228:refnum<class "MB_Master.lvclass">)  [unwired: 7 in]
                n105 = call "纳清蓝绿藻_第二点校准数据写入.vi"("error in (no error)"=w227, "数值"=w229, "MB session in"=w228) -> ("error out"=w221:errorcluster)  [unwired: 7 in, 1 out]
              }
              frame 3 {
                n106 = global read "多参数全局变量.vi" "MB session in"() -> (w234:refnum<class "MB_Master.lvclass">)
                n107 = call "纳清蓝绿藻_所有参数读取.vi"("MB session in"=w234) -> ("error out"=w232:errorcluster, "输出值"=w235:T6, "MB session out"=w233:refnum<class "MB_Master.lvclass">)  [unwired: 8 in]
                n108 = Unbundle By Name(w235) -> ("原始光强数值"=w236:u16)
                n109 = local read "标液3"() -> (w242:sgl)
                n110 = call "纳清蓝绿藻_第三点原始光强值写入.vi"("error in (no error)"=w232, "数值"=w236, "MB session in"=w233) -> ("error out"=w237:errorcluster, "MB session out"=w238:refnum<class "MB_Master.lvclass">)  [unwired: 7 in]
                n111 = call "纳清蓝绿藻_第三点校准数据写入.vi"("error in (no error)"=w237, "数值"=w242, "MB session in"=w238) -> ("error out"=w239:errorcluster, "MB session out"=w240:refnum<class "MB_Master.lvclass">)  [unwired: 7 in]
                n112 = call "纳清蓝绿藻_校准命令写入.vi"("error in (no error)"=w239, "数值"=u16 3 ("starting address"), "MB session in"=w240) -> ("error out"=w231:errorcluster)  [unwired: 7 in, 1 out]
              }
              frame 1, Default {
                n113 = global read "多参数全局变量.vi" "MB session in"() -> (w250:refnum<class "MB_Master.lvclass">)
                n114 = call "纳清蓝绿藻_所有参数读取.vi"("MB session in"=w250) -> ("error out"=w252:errorcluster, "输出值"=w249:T6, "MB session out"=w251:refnum<class "MB_Master.lvclass">)  [unwired: 8 in]
                n115 = Unbundle By Name(w249) -> ("原始光强数值"=w248:u16)
                n116 = local read "标液1"() -> (w245:sgl)
                n117 = call "纳清蓝绿藻_第一点原始光强值写入.vi"("error in (no error)"=w252, "数值"=w248, "MB session in"=w251) -> ("error out"=w247:errorcluster, "MB session out"=w246:refnum<class "MB_Master.lvclass">)  [unwired: 7 in]
                n118 = call "纳清蓝绿藻_第一点校准数据写入.vi"("error in (no error)"=w247, "数值"=w245, "MB session in"=w246) -> ("error out"=w244:errorcluster)  [unwired: 7 in, 1 out]
              }
            }
          }
        }
        n119 = case shown="1" w157 {
          tunnel: w160 -> [_ w167 w169 w171]
          tunnel: w159 -> [_ w166 w168 w170]
          frame 0, Default {
          }
          frame 1 {
            "第一点信号值" <- w167
            "第一点校准值" <- w166
          }
          frame 2 {
            "第二点信号值" <- w169
            "第二点校准值" <- w168
          }
          frame 3 {
            "第三点信号值" <- w171
            "第三点校准值" <- w170
          }
        }
        n120 = case shown="错误" w165 {
          tunnel: w164 -> [w173 _]
          tunnel: [w173 "Cal: Calibration failed" ("State(s) In (\"\")")] -> w161
          tunnel: w157 -> [w172 _]
          frame No Error {
            n121 = flat-sequence {
              tunnel: w172 -> [w174]
              frame #0 {
                n122 = Format Into String(format string="第%d点校准通过，按确认继续。" ("格式字符串"), w174) -> (resulting string=w176:string)  [unwired: 2 in, 1 out]
                n123 = One Button Dialog(message=w176) -> ()  [unwired: 1 in, 1 out]
              }
              frame #1 {
                n124 = Wait (ms)(milliseconds to wait=u32 2000 ("等待时间（毫秒）")) -> ()  [unwired: 1 out]
              }
            }
          }
          frame Error {
          }
        }
        n125 = call "Add State to Queue.vi"("State(s) In Front (\"\")"=w161, "State(s) In (\"\")"=w163) -> ("States Out"=w162:string)  [unwired: 13 in]
      }
      frame "Cal: Calibration failed" {
        n126 = global read "多参数全局变量.vi" "多参数编号"() -> (w258:string)
        n127 = call "Add State to Queue.vi"("State(s) In (\"\")"="init: all\nCal: Over\nidle" ("State(s) In (\"\")")) -> ("States Out"=w261:string)  [unwired: 14 in]
        n128 = Format Into String(format string="编号：%s\n参数：%s\n信息：%s" ("格式字符串"), w258, w255, "校准失败！" ("消息")) -> (resulting string=w257:string)  [unwired: 2 in, 1 out]
        n129 = One Button Dialog(message=w257) -> ()  [unwired: 1 in, 1 out]
        n130 = call "校准日志.vi"("table"="校准记录", "日志信息"=w257) -> ()  [unwired: 9 in, 1 out]
      }
      frame "Cal: Pass" {
        n131 = flat-sequence {
          tunnel: [w278] -> w268
          tunnel: w267 -> [w277]
          frame #0 {
            n132 = Wait (ms)(milliseconds to wait=u32 3000 ("等待时间（毫秒）")) -> ()  [unwired: 1 out]
          }
          frame #1 {
            n133 = case shown="2" w277 {
              tunnel: [w286 w297 w302] -> w278
              frame 0, Default {
                n134 = local read "第二点信号值"() -> (w280:dbl)
                n135 = local read "标液1"() -> (w282:sgl)
                n136 = local read "第一点校准值"() -> (w284:dbl)
                n137 = local read "第一点信号值"() -> (w285:dbl)
                n138 = local read "第二点校准值"() -> (w281:dbl)
                n139 = local read "标液2"() -> (w279:sgl)
                n140 = Format Into String(format string="校准结果：\n第一点校准值=%#.2f，第一点信号值=%#.2f，第一点标准值=%#.2f；\n第二点校准值=%#.2f，第二点信号值=%#.2f，第二点标准值=%#.2f。" ("提示"), w284, w285, w282, w281, w280, w279) -> (resulting string=w286:string)  [unwired: 2 in, 1 out]
              }
              frame 2 {
                n141 = local read "第三点信号值"() -> (w288:dbl)
                n142 = local read "第二点信号值"() -> (w291:dbl)
                n143 = local read "标液1"() -> (w293:sgl)
                n144 = local read "第三点校准值"() -> (w289:dbl)
                n145 = local read "标液3"() -> (w287:sgl)
                n146 = local read "第一点校准值"() -> (w295:dbl)
                n147 = local read "第一点信号值"() -> (w296:dbl)
                n148 = local read "第二点校准值"() -> (w292:dbl)
                n149 = local read "标液2"() -> (w290:sgl)
                n150 = Format Into String(format string="校准结果：\n第一点校准值=%#.2f，第一点信号值=%#.2f，第一点标准值=%#.2f；\n第二点校准值=%#.2f，第二点信号值=%#.2f，第二点标准值=%#.2f；\n第三点校准值=%#.2f，第三点信号值=%#.2f，第三点标准值=%#.2f。" ("提示"), w295, w296, w293, w292, w291, w290, w289, w288, w287) -> (resulting string=w297:string)  [unwired: 2 in, 1 out]
              }
              frame 1 {
                n151 = local read "第一点校准值"() -> (w301:dbl)
                n152 = local read "第一点信号值"() -> (w299:dbl)
                n153 = local read "标液1"() -> (w298:sgl)
                n154 = Format Into String(format string="校准结果：\n校准值=%#.2f，信号值=%#.2f，标准值=%#.2f。" ("提示"), w301, w299, w298) -> (resulting string=w302:string)  [unwired: 2 in, 1 out]
              }
            }
          }
        }
        n155 = call "Add State to Queue.vi"("State(s) In (\"\")"="init: all\nCal: Over\nidle" ("State(s) In (\"\")")) -> ("States Out"=w266:string)  [unwired: 14 in]
        n156 = global read "多参数全局变量.vi" "多参数编号"() -> (w272:string)
        n157 = Format Into String(format string="编号：%s\n参数：%s\n信息：%s" ("格式字符串"), w272, w271, w268) -> (resulting string=w269:string)  [unwired: 2 in, 1 out]
        n158 = One Button Dialog(message=w269) -> ()  [unwired: 1 in, 1 out]
        n159 = call "校准日志.vi"("table"="校准记录", "日志信息"=w269) -> ()  [unwired: 9 in, 1 out]
      }
      frame "Cal: Over" {
        n160 = global read "多参数全局变量.vi" "校准运行状态"() -> (w308:T7)
        n161 = Bundle By Name(cluster=w308, "藻密度"=FALSE ("Cond")) -> (w309:T7)
        n162 = global write "多参数全局变量.vi" "校准运行状态"(w309) -> ()
      }
      frame "idle", Default {
        n163 = event shown="[6] \"滤波设定\": 值改变" {
          selector: _ -> [_ _ _ _ _ _ _ _ _ _]
          dyn-events: _ -> [_ _ _ _ _ _ _ _ _ _]
          timeout: 10 -> [_ _ _ _ _ _ _ _ _ _]
          tunnel: w316 -> [w319 w323 w328 w331 w336 w341 w346 w354 w364 _]
          tunnel: [w318 w322 w329 w335 w340 w345 w348 w356 w363 w369] -> w315
          tunnel: [w317 w320 w330 w334 w339 w344 w347 w355 w361 w370] -> w314
          tunnel: w313 -> [w317 w320 w330 w334 w339 w344 w347 w355 w361 w370]
          tunnel: [_ _ _ _ _ _ _ _ w357 _] -> _
          event Timeout {
            n164 = event-data() -> ()  [unwired: 1 in, 3 out]
            n165 = call "Add State to Queue.vi"("State(s) In (\"\")"=w319) -> ("States Out"=w318:string)  [unwired: 14 in]
          }
          event "校准模式": Value Change {
            n166 = event-data() -> ()  [unwired: 1 in, 6 out]
            n167 = call "Add State to Queue.vi"("State(s) In (\"\")"=w323, "State(s) At Back (\"\")"="init: all\nidle" ("State(s) In (\"\")")) -> ("States Out"=w322:string)  [unwired: 13 in]
          }
          event "标液1", "标液2", "标液3", "滤波设定": Mouse Down {
            n168 = event-data() -> ("CtlRef"=w327:refnum<vi>)  [unwired: 1 in, 7 out]
            n169 = property class="DigNum (严格)"(reference=w327) -> (reference out=w324:refnum<vi>, "Value"=w325:sgl)  [unwired: 1 in, 1 out]
            n170 = call "数字键盘.vi"("OldNumber"=w325) -> ("NewNumber"=w326:dbl)  [unwired: 1 in]
            n171 = property class="DigNum (严格)"(reference=w324, "Val(Sgnl)"=w326) -> ()  [unwired: 1 in, 2 out]
            n172 = call "Add State to Queue.vi"("State(s) In (\"\")"=w328) -> ("States Out"=w329:string)  [unwired: 14 in]
          }
          event "标液1": Value Change {
            n173 = event-data() -> ("NewVal"=w332:sgl)  [unwired: 1 in, 5 out]
            n174 = global read "多参数全局变量.vi" "MB session in"() -> (w333:refnum<class "MB_Master.lvclass">)
            n175 = call "纳清蓝绿藻_第一点校准数据写入.vi"("数值"=w332, "MB session in"=w333) -> ()  [unwired: 8 in, 2 out]
            n176 = call "Add State to Queue.vi"("State(s) In (\"\")"=w331) -> ("States Out"=w335:string)  [unwired: 14 in]
          }
          event "标液2": Value Change {
            n177 = event-data() -> ("NewVal"=w337:sgl)  [unwired: 1 in, 5 out]
            n178 = global read "多参数全局变量.vi" "MB session in"() -> (w338:refnum<class "MB_Master.lvclass">)
            n179 = call "纳清蓝绿藻_第二点校准数据写入.vi"("数值"=w337, "MB session in"=w338) -> ()  [unwired: 8 in, 2 out]
            n180 = call "Add State to Queue.vi"("State(s) In (\"\")"=w336) -> ("States Out"=w340:string)  [unwired: 14 in]
          }
          event "标液3": Value Change {
            n181 = event-data() -> ("NewVal"=w342:sgl)  [unwired: 1 in, 5 out]
            n182 = global read "多参数全局变量.vi" "MB session in"() -> (w343:refnum<class "MB_Master.lvclass">)
            n183 = call "纳清蓝绿藻_第三点校准数据写入.vi"("数值"=w342, "MB session in"=w343) -> ()  [unwired: 8 in, 2 out]
            n184 = call "Add State to Queue.vi"("State(s) In (\"\")"=w341) -> ("States Out"=w345:string)  [unwired: 14 in]
          }
          event "滤波设定": Value Change {
            n185 = event-data() -> ()  [unwired: 1 in, 6 out]
            n186 = flat-sequence {
              frame #0 {
                n187 = global read "断电保存变量.vi" "滤波设置"() -> (w351:T3)
                n188 = local read "滤波设定"() -> (w349:sgl)
                n189 = Bundle By Name(cluster=w351, "藻密度"=w349) -> (w350:T3)
                n190 = global write "断电保存变量.vi" "滤波设置"(w350) -> ()
              }
              frame #1 {
                n191 = call "配置文件保存.vi"() -> ()  [unwired: 12 in]
              }
            }
            n192 = call "Add State to Queue.vi"("State(s) In (\"\")"=w346) -> ("States Out"=w348:string)  [unwired: 14 in]
          }
          event "量程": Value Change {
            n193 = event-data() -> ("NewVal"=w352:u16)  [unwired: 1 in, 5 out]
            n194 = global read "多参数全局变量.vi" "MB session in"() -> (w353:refnum<class "MB_Master.lvclass">)
            n195 = call "纳清蓝绿藻_量程写入.vi"("数值"=w352, "MB session in"=w353) -> ()  [unwired: 8 in, 2 out]
            n196 = call "Add State to Queue.vi"("State(s) In (\"\")"=w354) -> ("States Out"=w356:string)  [unwired: 14 in]
          }
          event "校准启动": Value Change {
            n197 = event-data() -> ()  [unwired: 1 in, 6 out]
            n198 = global read "纳清过程全局变量.vi" "蓝绿藻测试值"() -> (w359:T2)
            n199 = Unbundle By Name(w359) -> ("量程"=w358:u16)
            n200 = global read "多参数全局变量.vi" "MB session in"() -> (w360:refnum<class "MB_Master.lvclass">)
            n201 = call "纳清蓝绿藻_校准量程写入.vi"("数值"=w358, "MB session in"=w360) -> ("error out"=w357:errorcluster)  [unwired: 8 in, 1 out]
            n202 = call "Add State to Queue.vi"("State(s) In (\"\")"=w364, "State(s) At Back (\"\")"="init: all\nCal: Place standard solution\n Cal: Calibration process\nidle" ("State(s) In (\"\")")) -> ("States Out"=w363:string)  [unwired: 13 in]
          }
          event "校准停止": Value Change {
            n203 = event-data() -> ()  [unwired: 1 in, 6 out]
            n204 = global read "多参数全局变量.vi" "校准运行状态"() -> (w366:T7)
            n205 = Bundle By Name(cluster=w366, "藻密度"=TRUE ("Cond")) -> (w367:T7)
            n206 = global write "多参数全局变量.vi" "校准运行状态"(w367) -> ()
            n207 = call "Add State to Queue.vi"("State(s) In (\"\")"="init: all\nCal: Over\nidle" ("State(s) In (\"\")")) -> ("States Out"=w369:string)  [unwired: 14 in]
          }
        }
      }
    }
  }
